vi "initialise task.vi"(8 "error in (no error)":errorcluster, 11 "ImagingModeSPIM in":refnum<class "ImagingModeSPIM.lvclass">) -> (0 "error out":errorcluster, 3 "ImagingModeSPIM out":refnum<class "ImagingModeSPIM.lvclass">)   [LabVIEW 2012, in "ImagingModeSPIM.lvclass"]
uses:
  ImagingModeSPIM.lvclass
  ImagingModeSPIM.lvclass/ImagingModeSPIM.ctl
  <vilib>/DAQmx/write.llb/DAQmx Write (Analog DBL 1Chan 1Samp).vi
  <vilib>/DAQmx/create/channels.llb/DAQmx Create Channel (AO-Voltage-Basic).vi
  <vilib>/DAQmx/miscellaneous.llb/DAQmx Fill In Error Info.vi
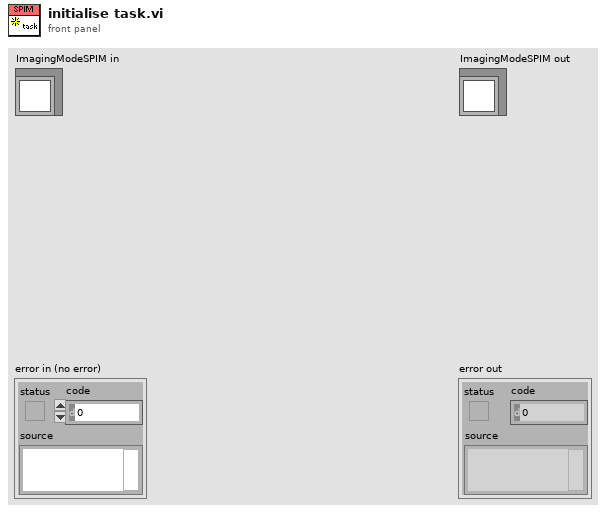
[diagram p1: front panel]
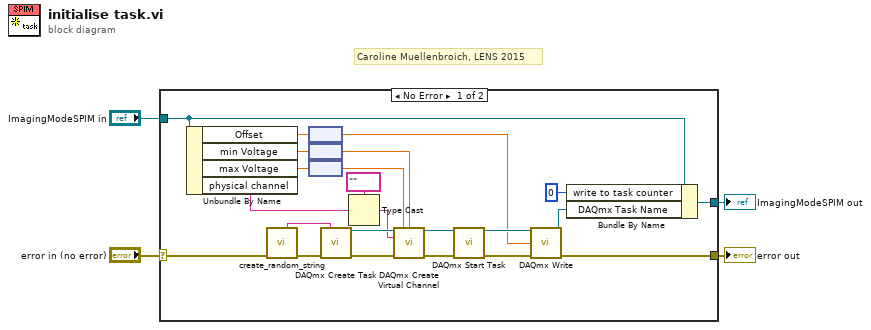
[diagram p0: block diagram]
diagram:
  # "Caroline Muellenbroich, LENS 2015"
  n1 = case shown="No Error" "error in (no error)" {
    selector: "error in (no error)" -> [w9 w29]
    tunnel: [w16 w29] -> w3
    tunnel: [w26 w28] -> w1
    tunnel: "ImagingModeSPIM in" -> [w27 w28]
    frame No Error {
      n2 = Unbundle By Name(w27) -> ("Offset"=w15:dbl[unit], "min Voltage"=w24:dbl[unit], "max Voltage"=w25:dbl[unit], "physical channel"=w23:string)
      n3 = call "create_random_string.vi"("error in (no error)"=w9) -> ("error out"=w8:errorcluster, "random string"=w5:string)  [unwired: 9 in]
      n4 = node(w15) -> (w14:dbl)
      n5 = node(w24) -> (w7:dbl)
      n6 = node(w25) -> (w6:dbl)
      n7 = call <vilib>:"DAQmx Create Task.vi"("new task name"=w5, "error in"=w8) -> ("task out"=w12:refnum<k21>, "error out"=w13:errorcluster)  [unwired: 12 in]
      n8 = Type Cast(type=tag "" ("physical channels"), x=w23) -> (*(type *) &x=w10:tag)
      n9 = call-poly <vilib>:"DAQmx Create Virtual Channel.vi"("task in"=w12, "maximum value"=w6, "minimum value"=w7, "physical channels"=w10, "error in"=w13) -> ("task out"=w20:refnum<k21>, "error out"=w22:errorcluster)  [unwired: 9 in]
      n10 = call <vilib>:"DAQmx Start Task.vi"("task/channels in"=w20, "error in"=w22) -> ("task out"=w17:refnum<k21>, "error out"=w18:errorcluster)  [unwired: 12 in]
      n11 = call-poly <vilib>:"DAQmx Write.vi"("task/channels in"=w17, "data"=w14, "error in"=w18) -> ("task out"=w19:refnum<k21>, "error out"=w16:errorcluster)  [unwired: 10 in, 1 out]
      n12 = Bundle By Name(cluster=w27, "write to task counter"=0 ("runtime cluster.Task cluster.write to task counter"), "DAQmx Task Name"=w19) -> (w26:refnum<class "ImagingModeSPIM.lvclass">)
    }
    frame Error {
    }
  }
  "error out" <- w3
  "ImagingModeSPIM out" <- w1
